vi "create_zero_centered.vi"(6 "z dimension":dbl[unit], 8 "error in (no error)":errorcluster, 9 "y dimension":dbl[unit], 10 "x dimension":dbl[unit]) -> (0 "error out":errorcluster, 3 "Box out":refnum<class "Box.lvclass">)   [LabVIEW 2010, in "Box.lvclass"]
uses:
  Box.lvclass
  SpaceVector/SpaceVector/SpaceVector.lvclass
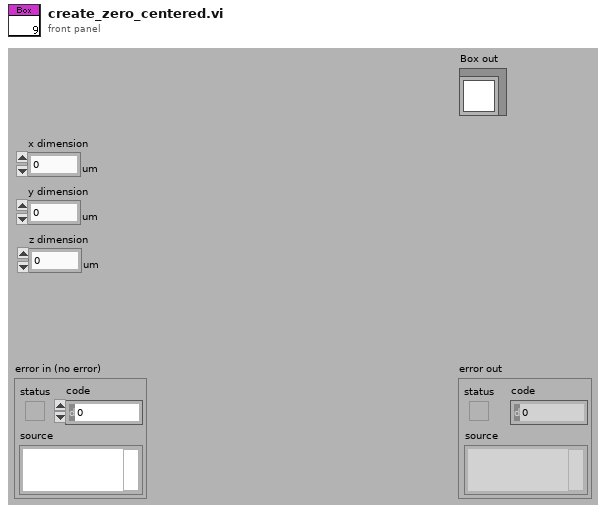
[diagram p1: front panel]
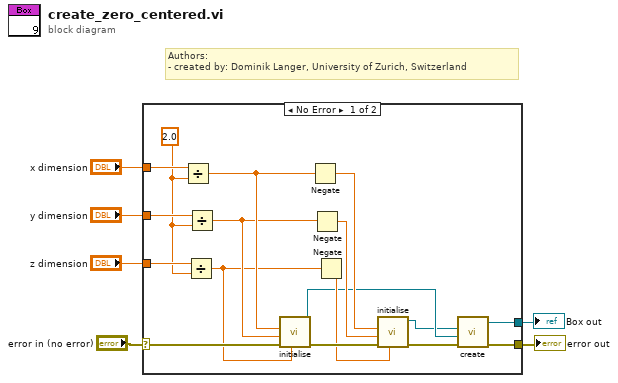
[diagram p0: block diagram]
diagram:
  # "Authors: \n- created by: Dominik Langer, University of Zurich, Switzerland"
  n1 = case shown="No Error" "error in (no error)" {
    selector: "error in (no error)" -> [w19 w24]
    tunnel: [w13 w24] -> w5
    tunnel: [w12 _] -> w4
    tunnel: "x dimension" -> [w23 _]
    tunnel: "y dimension" -> [w22 _]
    tunnel: "z dimension" -> [w21 _]
    frame No Error {
      w20 = 2.0
      n2 = Divide(x=w23, y=w20) -> (x/y=w18:dbl[unit])
      n3 = Divide(x=w21, y=w20) -> (x/y=w16:dbl[unit])
      n4 = Divide(x=w22, y=w20) -> (x/y=w17:dbl[unit])
      n5 = call "initialise.vi"("z"=w16, "error in (no error)"=w19, "y"=w17, "x"=w18) -> ("error out"=w15:errorcluster, "SpaceVector out"=w8:refnum<class "SpaceVector.lvclass">)  [unwired: 6 out]
      n6 = Negate(x=w18) -> (-x=w11:dbl[unit])
      n7 = Negate(x=w17) -> (-x=w10:dbl[unit])
      n8 = Negate(x=w16) -> (-x=w9:dbl[unit])
      n9 = call "initialise.vi"("z"=w9, "error in (no error)"=w15, "y"=w10, "x"=w11) -> ("error out"=w14:errorcluster, "SpaceVector out"=w7:refnum<class "SpaceVector.lvclass">)  [unwired: 6 out]
      n10 = call "create.vi"("error in (no error)"=w14, "maximum"=w8, "minimum"=w7) -> ("error out"=w13:errorcluster, "Box out"=w12:refnum<class "Box.lvclass">)  [unwired: 7 out]
    }
    frame Error {
    }
  }
  "error out" <- w5
  "Box out" <- w4
